vi "Read RP I-V Configuration.vi"(8 "error in (no error)":errorcluster, 11 "RP I-V in":refnum<class "RP I-V.lvclass">) -> (0 "error out":errorcluster, 2 "Configuration":T1={"I-V parameters"={"Start magnitude"=0.0, "Magnitude increment"=0.0, "End magnitude"=0.0, "Ramp length"=0, "Top  length"=0, "Threshold "=0.0, "Processing delay"=0, "Valhalla range"=0.0, "Interpolation"=0, "Stop after"=1, "Detector window"=480}, "Ranges"=[1.0, 1.0], "Pre-trigger duration"=0.01, "Post-trigger duration"=0.1, "Output delay"=0.1} {"Output delay" format="%#_6ps"; "Post-trigger duration" format="%#_6ps"; "Pre-trigger duration" format="%#_6ps"; "Ranges" format="%#_6pV"; "I-V parameters"."Detector window" format="%dpts"; "I-V parameters"."Stop after" format="%d sweep(s)"; "I-V parameters"."Valhalla range" format="%#_6pA"; "I-V parameters"."Processing delay" format="%dpts"; "I-V parameters"."Threshold" format="%#_6pV"; "I-V parameters"."Top  length" format="%dpts"; "I-V parameters"."Ramp length" format="%dpts"; "I-V parameters"."End magnitude" format="%#_6pA"; "I-V parameters"."Magnitude increment" format="%#_6pA"; "I-V parameters"."Start magnitude" format="%#_6pA"}, 3 "RP I-V out":refnum<class "RP I-V.lvclass">)   [LabVIEW 2016, in "RP I-V.lvclass"]
uses:
  RP I-V.lvclass
  C:/github/LabActor/Template Module/Template Module.lvclass
  NHMFL_Core/Libraries/Red Pitaya/RP Core/Rep Pitaya I-V driver/RP I-V Configuration.ctl
  NHMFL_Core/Libraries/Red Pitaya/Waform generation/I-V parameters.ctl
  Template Module/Template Module.lvclass/Template Module.ctl
  Template Module/Read Configuration.vi
panel:
  # "Waveform parameters"
  # "Detector parameters"
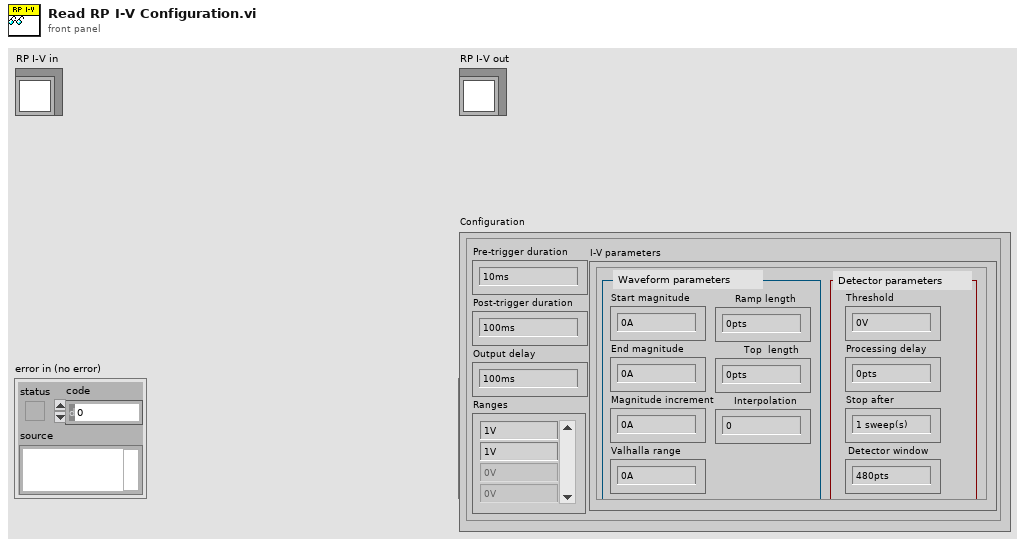
[diagram p1: front panel]
types:
  T1 = typedef "RP I-V Configuration.ctl" = cluster{"I-V parameters":T2, "Ranges":dbl[], "Pre-trigger duration":dbl, "Post-trigger duration":dbl, "Output delay":dbl}
  T2 = typedef "I-V parameters.ctl" = cluster{"Start magnitude":dbl, "Magnitude increment":dbl, "End magnitude":dbl, "Ramp length":i32, "Top  length":i32, "Threshold ":dbl, "Processing delay":u16, "Valhalla range":dbl, "Interpolation":i32, "Stop after":u16, "Detector window":i32}
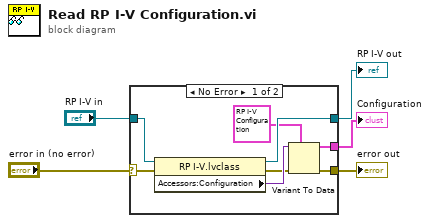
[diagram p0: block diagram]
diagram:
  n1 = case shown="No Error" "error in (no error)" {
    selector: "error in (no error)" -> [w7 w14]
    tunnel: [w6 w14] -> w2
    tunnel: [w10 w15] -> w5
    tunnel: "RP I-V in" -> [w11 w15]
    tunnel: [w8 _] -> w1
    frame No Error {
      n2 = property class="RP I-V.lvclass"(reference=w11, error in=w7) -> (reference out=w10:refnum<class "RP I-V.lvclass">, error out=w12:errorcluster, "Accessors:Configuration"=w13:variant)
      n3 = Variant To Data(error in=w12, type=T1 {"I-V parameters"={"Start magnitude"=0.0, "Magnitude increment"=0.0, "End magnitude"=0.0, "Ramp length"=0, "Top  length"=0, "Threshold "=0.0, "Processing delay"=0, "Valhalla range"=0.0, "Interpolation"=0, "Stop after"=1, "Detector window"=480}, "Ranges"=[1.0, 1.0], "Pre-trigger duration"=0.01, "Post-trigger duration"=0.1, "Output delay"=0.1} ("Configuration"), Variant=w13) -> (data=w8:T1, error out=w6:errorcluster)
    }
    frame Error {
    }
  }
  "error out" <- w2
  "RP I-V out" <- w5
  "Configuration" <- w1
